vi "Mangle.vi"(1 "String In":string) -> (0 "String Out":string)   [LabVIEW 2020, in "Configit.lvlib"]
uses:
  Configit.lvlib
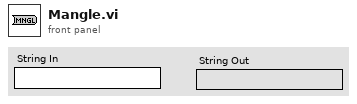
[diagram p1: front panel]
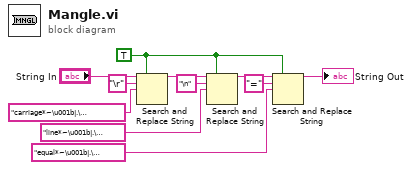
[diagram p0: block diagram]
diagram:
  w7 = TRUE ("replace all? (F)")
  n1 = Search and Replace String(replace all?=w7, input string="String In", search string="\r" ("replace string (\"\")"), replace string="carriage*~\u001b|.\u0017return") -> (result string=w10:string)  [unwired: 4 in, 3 out]
  n2 = Search and Replace String(replace all?=w7, input string=w10, search string="\n" ("replace string (\"\")"), replace string="line*~\u001b|.\u0017feed") -> (result string=w9:string)  [unwired: 4 in, 3 out]
  n3 = Search and Replace String(replace all?=w7, input string=w9, search string="=" ("replace string (\"\")"), replace string="equal*~\u001b|.\u0017sign") -> (result string=→"String Out":string)  [unwired: 4 in, 3 out]
